vi "HEWH RLT PRAT.vi"() -> ()   [LabVIEW 2016] (continued)
              tunnel: w3221 -> [w3243 _]
              tunnel: w3220 -> [w3244 _]
              tunnel: w3218 -> [w3242 _]
              tunnel: w3217 -> [w3241 _]
              tunnel: w3215 -> [w3239 _]
              tunnel: w3210 -> [w3238 _]
              frame False {
                n1364 = Generate User Event(user event=w3250, event data cluster=TRUE ("event data"), error in=w3249) -> (error out=w3247:errorcluster)  [unwired: 1 in, 1 out]
                n1365 = local write "StationD Setpoint"(w3239) -> ()
                n1366 = local write "Disable Station 4"(HEWH_RLT_Station_Disable."Enable Station" ("Disable Station 4")) -> ()
                n1367 = local write "Cutout Delay D (sec)"(w3241) -> ()
                n1368 = Generate User Event(user event=w3245, event data cluster=TRUE ("event data"), error in=w3247) -> (error out=w3246:errorcluster)  [unwired: 1 in, 1 out]
                "Station D Test Sequence" <- w3253
                "Station ID to Reset" <- w3252
                "Appliance Details D" <- w3244
                "Updated File Path D" <- w3243
                "Log Data Output (D)" <- w3242
                "Test Procedure 4" <- w3238
              }
              frame True {
              }
            }
          }
          event "DAQ for A": Value Change {
            n1369 = event-data() -> ("NewVal"=w3255:bool)  [unwired: 1 in, 5 out]
            n1370 = case shown="True" w3255 {
              frame False {
                w3259 = T67."Enabled" ("Disabled")
                n1371 = property on="DAQ for A" class="Bool (strict)"("DisabledEnum"=w3259) -> ()  [unwired: 2 in, 2 out]
                n1372 = property on="DAQ for B" class="Bool (strict)"("DisabledEnum"=w3259) -> ()  [unwired: 2 in, 2 out]
                n1373 = property on="DAQ for C" class="Bool (strict)"("DisabledEnum"=w3259) -> ()  [unwired: 2 in, 2 out]
                n1374 = property on="DAQ for D" class="Bool (strict)"("DisabledEnum"=w3259) -> ()  [unwired: 2 in, 2 out]
              }
              frame True {
                w3261 = T67."Disabled and Grayed Out" ("Disabled")
                n1375 = property on="DAQ for D" class="Bool (strict)"("DisabledEnum"=w3261) -> ()  [unwired: 2 in, 2 out]
                n1376 = property on="DAQ for B" class="Bool (strict)"("DisabledEnum"=w3261) -> ()  [unwired: 2 in, 2 out]
                n1377 = property on="DAQ for C" class="Bool (strict)"("DisabledEnum"=w3261) -> ()  [unwired: 2 in, 2 out]
                n1378 = property on="DAQ for A" class="Bool (strict)"("DisabledEnum"=T67."Enabled" ("Disabled")) -> ()  [unwired: 2 in, 2 out]
              }
            }
          }
          event "DAQ for B": Value Change {
            n1379 = event-data() -> ("NewVal"=w3262:bool)  [unwired: 1 in, 5 out]
            n1380 = case shown="True" w3262 {
              frame False {
                w3266 = T67."Enabled" ("Disabled")
                n1381 = property on="DAQ for A" class="Bool (strict)"("DisabledEnum"=w3266) -> ()  [unwired: 2 in, 2 out]
                n1382 = property on="DAQ for B" class="Bool (strict)"("DisabledEnum"=w3266) -> ()  [unwired: 2 in, 2 out]
                n1383 = property on="DAQ for C" class="Bool (strict)"("DisabledEnum"=w3266) -> ()  [unwired: 2 in, 2 out]
                n1384 = property on="DAQ for D" class="Bool (strict)"("DisabledEnum"=w3266) -> ()  [unwired: 2 in, 2 out]
              }
              frame True {
                w3267 = T67."Disabled and Grayed Out" ("Disabled")
                n1385 = property on="DAQ for A" class="Bool (strict)"("DisabledEnum"=w3267) -> ()  [unwired: 2 in, 2 out]
                n1386 = property on="DAQ for C" class="Bool (strict)"("DisabledEnum"=w3267) -> ()  [unwired: 2 in, 2 out]
                n1387 = property on="DAQ for D" class="Bool (strict)"("DisabledEnum"=w3267) -> ()  [unwired: 2 in, 2 out]
                n1388 = property on="DAQ for B" class="Bool (strict)"("DisabledEnum"=T67."Enabled" ("Disabled")) -> ()  [unwired: 2 in, 2 out]
              }
            }
          }
          event "DAQ for C": Value Change {
            n1389 = event-data() -> ("NewVal"=w3269:bool)  [unwired: 1 in, 5 out]
            n1390 = case shown="True" w3269 {
              frame False {
                w3273 = T67."Enabled" ("Disabled")
                n1391 = property on="DAQ for A" class="Bool (strict)"("DisabledEnum"=w3273) -> ()  [unwired: 2 in, 2 out]
                n1392 = property on="DAQ for B" class="Bool (strict)"("DisabledEnum"=w3273) -> ()  [unwired: 2 in, 2 out]
                n1393 = property on="DAQ for C" class="Bool (strict)"("DisabledEnum"=w3273) -> ()  [unwired: 2 in, 2 out]
                n1394 = property on="DAQ for D" class="Bool (strict)"("DisabledEnum"=w3273) -> ()  [unwired: 2 in, 2 out]
              }
              frame True {
                w3274 = T67."Disabled and Grayed Out" ("Disabled")
                n1395 = property on="DAQ for A" class="Bool (strict)"("DisabledEnum"=w3274) -> ()  [unwired: 2 in, 2 out]
                n1396 = property on="DAQ for B" class="Bool (strict)"("DisabledEnum"=w3274) -> ()  [unwired: 2 in, 2 out]
                n1397 = property on="DAQ for D" class="Bool (strict)"("DisabledEnum"=w3274) -> ()  [unwired: 2 in, 2 out]
                n1398 = property on="DAQ for C" class="Bool (strict)"("DisabledEnum"=T67."Enabled" ("Disabled")) -> ()  [unwired: 2 in, 2 out]
              }
            }
          }
          event "DAQ for D": Value Change {
            n1399 = event-data() -> ("NewVal"=w3276:bool)  [unwired: 1 in, 5 out]
            n1400 = case shown="True" w3276 {
              frame False {
                w3280 = T67."Enabled" ("Disabled")
                n1401 = property on="DAQ for A" class="Bool (strict)"("DisabledEnum"=w3280) -> ()  [unwired: 2 in, 2 out]
                n1402 = property on="DAQ for B" class="Bool (strict)"("DisabledEnum"=w3280) -> ()  [unwired: 2 in, 2 out]
                n1403 = property on="DAQ for C" class="Bool (strict)"("DisabledEnum"=w3280) -> ()  [unwired: 2 in, 2 out]
                n1404 = property on="DAQ for D" class="Bool (strict)"("DisabledEnum"=w3280) -> ()  [unwired: 2 in, 2 out]
              }
              frame True {
                w3282 = T67."Disabled and Grayed Out" ("Disabled")
                n1405 = property on="DAQ for A" class="Bool (strict)"("DisabledEnum"=w3282) -> ()  [unwired: 2 in, 2 out]
                n1406 = property on="DAQ for B" class="Bool (strict)"("DisabledEnum"=w3282) -> ()  [unwired: 2 in, 2 out]
                n1407 = property on="DAQ for C" class="Bool (strict)"("DisabledEnum"=w3282) -> ()  [unwired: 2 in, 2 out]
                n1408 = property on="DAQ for D" class="Bool (strict)"("DisabledEnum"=T67."Enabled" ("Disabled")) -> ()  [unwired: 2 in, 2 out]
              }
            }
          }
          event "Set Valves": Value Change {
            n1409 = event-data() -> ("NewVal"=w3284:bool)  [unwired: 1 in, 5 out]
            n1410 = call "UTILITY Aquire Semaphore.vi"("error in (no error)"=w3291, "Refnum in"=w3288) -> ("error out"=w3283:errorcluster, "Refnum out"=w3287:T56)  [unwired: 7 in, 1 out]
            n1411 = case shown="True" w3284 {
              tunnel: w3283 -> [w3292 w3299]
              tunnel: [w3292 w3298] -> w3289
              tunnel: w3286 -> [_ w3294]
              frame False {
              }
              frame True {
                n1412 = Unbundle By Name(w3294) -> ("Test Fixture Hardware.Analog Data.Yokogawa.MW100"=w3295:refnum<visa-resource-name>)
                n1413 = local read "Pressurize Tank?"() -> (w3296:bool)
                n1414 = call "HEWH Solenoid Bank.vi"("VISA session"=w3295, "Valve Bank Setting"="Valve Bank Setting", "Station ID"="Station ID", "Pressurize Tank?"=w3296, "Error In"=w3299, "Debug"=TRUE) -> ("Error Out"=w3298:errorcluster)  [unwired: 8 in, 1 out]
              }
            }
            n1415 = call "UTILITY Release Semaphore.vi"("error in (no error)"=w3289, "Refnum in"=w3287) -> ("error out"=w3290:errorcluster)  [unwired: 9 in]
          }
          event "Send GEA CMD": Value Change {
            n1416 = event-data() -> ()  [unwired: 1 in, 6 out]
            n1417 = local read "Station ID"() -> (w3309:T25)
            n1418 = call "HEWH_DSM_CMD.vi"("Heating Mode"="Heating Mode", "GEA2 Commands and Requests"=GEA2_Commands."CMD_UPDATE_MODE") -> ("Input Data"=w3312:T74)  [unwired: 7 in, 1 out]
            n1419 = call "HEWH_DSM_CMD.vi"("Temperature"="Unit Setpoint", "GEA2 Commands and Requests"=GEA2_Commands."CMD_WRITE_SETPOINTS") -> ("Input Data"=w3311:T74)  [unwired: 7 in, 1 out]
            n1420 = case shown="\"A\"" w3309 {
              tunnel: w3313 -> [w3320 w3328 w3347 w3368 w3389]
              tunnel: w3312 -> [_ w3327 w3344 w3365 w3386]
              tunnel: w3311 -> [_ w3324 w3345 w3366 w3387]
              tunnel: [w3320 w3323 w3346 w3367 w3388] -> w3310
              tunnel: w3308 -> [_ _ _ _ w3384]
              tunnel: w3307 -> [_ _ _ _ w3385]
              tunnel: w3306 -> [_ _ _ w3363 _]
              tunnel: w3305 -> [_ _ _ w3364 _]
              tunnel: w3304 -> [_ _ w3343 _ _]
              tunnel: w3303 -> [_ _ w3342 _ _]
              tunnel: w3302 -> [_ w3321 _ _ _]
              tunnel: w3301 -> [_ w3322 _ _ _]
              frame "", Default {
              }
              frame "A" {
                n1421 = for {
                  N: 5 -> [_]
                  tunnel: w3322 -> [w3341]
                  tunnel: w3321 -> [w3340]
                  tunnel: w3327 -> [w3337]
                  shift-right: [w3338] -> w3325
                  shift-left: w3328 -> [w3339]
                  n1422 = call "GEA2 Send and Receive Message.vi"("GEA2 Reference In"=w3341, "Input Data"=w3337, "GEA2 Event Registration"=w3340, "Error In"=w3339) -> ("Error Out"=w3338:errorcluster)  [unwired: 6 in, 5 out]
                  n1423 = Wait Until Next ms Multiple(millisecond multiple=u32 100) -> ()  [unwired: 1 out]
                }
                n1424 = for {
                  N: 5 -> [_]
                  tunnel: w3322 -> [w3335]
                  tunnel: w3321 -> [w3334]
                  tunnel: w3324 -> [w3331]
                  shift-right: [w3332] -> w3323
                  shift-left: w3325 -> [w3333]
                  n1425 = call "GEA2 Send and Receive Message.vi"("GEA2 Reference In"=w3335, "Input Data"=w3331, "GEA2 Event Registration"=w3334, "Error In"=w3333) -> ("Error Out"=w3332:errorcluster)  [unwired: 6 in, 5 out]
                  n1426 = Wait Until Next ms Multiple(millisecond multiple=u32 100) -> ()  [unwired: 1 out]
                }
              }
              frame "B" {
                n1427 = for {
                  N: 5 -> [_]
                  tunnel: w3342 -> [w3362]
                  tunnel: w3343 -> [w3361]
                  tunnel: w3344 -> [w3358]
                  shift-right: [w3359] -> w3348
                  shift-left: w3347 -> [w3360]
                  n1428 = call "GEA2 Send and Receive Message.vi"("GEA2 Reference In"=w3362, "Input Data"=w3358, "GEA2 Event Registration"=w3361, "Error In"=w3360) -> ("Error Out"=w3359:errorcluster)  [unwired: 6 in, 5 out]
                  n1429 = Wait Until Next ms Multiple(millisecond multiple=u32 100) -> ()  [unwired: 1 out]
                }
                n1430 = for {
                  N: 5 -> [_]
                  tunnel: w3342 -> [w3356]
                  tunnel: w3343 -> [w3355]
                  tunnel: w3345 -> [w3352]
                  shift-right: [w3353] -> w3346
                  shift-left: w3348 -> [w3354]
                  n1431 = call "GEA2 Send and Receive Message.vi"("GEA2 Reference In"=w3356, "Input Data"=w3352, "GEA2 Event Registration"=w3355, "Error In"=w3354) -> ("Error Out"=w3353:errorcluster)  [unwired: 6 in, 5 out]
                  n1432 = Wait Until Next ms Multiple(millisecond multiple=u32 100) -> ()  [unwired: 1 out]
                }
              }
              frame "C" {
                n1433 = for {
                  N: 5 -> [_]
                  tunnel: w3364 -> [w3383]
                  tunnel: w3363 -> [w3382]
                  tunnel: w3365 -> [w3379]
                  shift-right: [w3380] -> w3369
                  shift-left: w3368 -> [w3381]
                  n1434 = call "GEA2 Send and Receive Message.vi"("GEA2 Reference In"=w3383, "Input Data"=w3379, "GEA2 Event Registration"=w3382, "Error In"=w3381) -> ("Error Out"=w3380:errorcluster)  [unwired: 6 in, 5 out]
                  n1435 = Wait Until Next ms Multiple(millisecond multiple=u32 100) -> ()  [unwired: 1 out]
                }
                n1436 = for {
                  N: 5 -> [_]
                  tunnel: w3364 -> [w3377]
                  tunnel: w3363 -> [w3376]
                  tunnel: w3366 -> [w3373]
                  shift-right: [w3374] -> w3367
                  shift-left: w3369 -> [w3375]
                  n1437 = call "GEA2 Send and Receive Message.vi"("GEA2 Reference In"=w3377, "Input Data"=w3373, "GEA2 Event Registration"=w3376, "Error In"=w3375) -> ("Error Out"=w3374:errorcluster)  [unwired: 6 in, 5 out]
                  n1438 = Wait Until Next ms Multiple(millisecond multiple=u32 100) -> ()  [unwired: 1 out]
                }
              }
              frame "D" {
                n1439 = for {
                  N: 5 -> [_]
                  tunnel: w3385 -> [w3404]
                  tunnel: w3384 -> [w3403]
                  tunnel: w3386 -> [w3400]
                  shift-right: [w3401] -> w3390
                  shift-left: w3389 -> [w3402]
                  n1440 = call "GEA2 Send and Receive Message.vi"("GEA2 Reference In"=w3404, "Input Data"=w3400, "GEA2 Event Registration"=w3403, "Error In"=w3402) -> ("Error Out"=w3401:errorcluster)  [unwired: 6 in, 5 out]
                  n1441 = Wait Until Next ms Multiple(millisecond multiple=u32 100) -> ()  [unwired: 1 out]
                }
                n1442 = for {
                  N: 5 -> [_]
                  tunnel: w3385 -> [w3398]
                  tunnel: w3384 -> [w3397]
                  tunnel: w3387 -> [w3394]
                  shift-right: [w3395] -> w3388
                  shift-left: w3390 -> [w3396]
                  n1443 = call "GEA2 Send and Receive Message.vi"("GEA2 Reference In"=w3398, "Input Data"=w3394, "GEA2 Event Registration"=w3397, "Error In"=w3396) -> ("Error Out"=w3395:errorcluster)  [unwired: 6 in, 5 out]
                  n1444 = Wait Until Next ms Multiple(millisecond multiple=u32 100) -> ()  [unwired: 1 out]
                }
              }
            }
          }
          event "X-Axis - Station A", "Y-Axis1 - Station A", "Y-Axis2 - Station A": Value Change {
            n1445 = event-data() -> ()  [unwired: 1 in, 6 out]
            n1446 = local read "Station A"() -> (w3409:string[][])
            n1447 = Transpose 2D Array(2D array=w3409) -> (transposed array=w3406:string[][])
            n1448 = Index Array(array=w3406, index (row)=0 ("disabled index (col)")) -> (element=w3412:string[])  [unwired: 1 in]
            n1449 = Index Array(array=w3406, index (row)=0 ("disabled index (col)")) -> (element=w3411:string[])  [unwired: 1 in]
            n1450 = Index Array(array=w3406, index (row)=0 ("disabled index (col)")) -> (element=w3410:string[])  [unwired: 1 in]
            n1451 = property on="X-Axis - Station A" class="CmbBox"("Strings[]"=w3412) -> ()  [unwired: 2 in, 2 out]
            n1452 = property on="Y-Axis2 - Station A" class="CmbBox"("Strings[]"=w3410) -> ()  [unwired: 2 in, 2 out]
            n1453 = property on="Y-Axis1 - Station A" class="CmbBox"("Strings[]"=w3411) -> ()  [unwired: 2 in, 2 out]
          }
          event "Y-Axis1 - Station B", "X-Axis - Station B", "Y-Axis2 - Station B": Value Change {
            n1454 = event-data() -> ()  [unwired: 1 in, 6 out]
            n1455 = local read "Station B"() -> (w3420:string[][])
            n1456 = Transpose 2D Array(2D array=w3420) -> (transposed array=w3419:string[][])
            n1457 = Index Array(array=w3419, index (row)=0 ("disabled index (col)")) -> (element=w3423:string[])  [unwired: 1 in]
            n1458 = Index Array(array=w3419, index (row)=0 ("disabled index (col)")) -> (element=w3422:string[])  [unwired: 1 in]
            n1459 = Index Array(array=w3419, index (row)=0 ("disabled index (col)")) -> (element=w3421:string[])  [unwired: 1 in]
            n1460 = property on="X-Axis - Station B" class="CmbBox"("Strings[]"=w3423) -> ()  [unwired: 2 in, 2 out]
            n1461 = property on="Y-Axis1 - Station B" class="CmbBox"("Strings[]"=w3422) -> ()  [unwired: 2 in, 2 out]
            n1462 = property on="Y-Axis2 - Station B" class="CmbBox"("Strings[]"=w3421) -> ()  [unwired: 2 in, 2 out]
          }
          event "X-Axis - Station C", "Y-Axis1 - Station C", "Y-Axis2 - Station C": Value Change {
            n1463 = event-data() -> ()  [unwired: 1 in, 6 out]
            n1464 = local read "Station C"() -> (w3431:string[][])
            n1465 = Transpose 2D Array(2D array=w3431) -> (transposed array=w3430:string[][])
            n1466 = Index Array(array=w3430, index (row)=0 ("disabled index (col)")) -> (element=w3434:string[])  [unwired: 1 in]
            n1467 = Index Array(array=w3430, index (row)=0 ("disabled index (col)")) -> (element=w3433:string[])  [unwired: 1 in]
            n1468 = Index Array(array=w3430, index (row)=0 ("disabled index (col)")) -> (element=w3432:string[])  [unwired: 1 in]
            n1469 = property on="X-Axis - Station C" class="CmbBox"("Strings[]"=w3434) -> ()  [unwired: 2 in, 2 out]
            n1470 = property on="Y-Axis1 - Station C" class="CmbBox"("Strings[]"=w3433) -> ()  [unwired: 2 in, 2 out]
            n1471 = property on="Y-Axis2 - Station C" class="CmbBox"("Strings[]"=w3432) -> ()  [unwired: 2 in, 2 out]
          }
          event "X-Axis - Station D", "Y-Axis1 - Station D", "Y-Axis2 - Station D": Value Change {
            n1472 = event-data() -> ()  [unwired: 1 in, 6 out]
            n1473 = local read "Station D"() -> (w3441:string[][])
            n1474 = Transpose 2D Array(2D array=w3441) -> (transposed array=w3442:string[][])
            n1475 = Index Array(array=w3442, index (row)=0 ("disabled index (col)")) -> (element=w3445:string[])  [unwired: 1 in]
            n1476 = Index Array(array=w3442, index (row)=0 ("disabled index (col)")) -> (element=w3444:string[])  [unwired: 1 in]
            n1477 = Index Array(array=w3442, index (row)=0 ("disabled index (col)")) -> (element=w3443:string[])  [unwired: 1 in]
            n1478 = property on="X-Axis - Station D" class="CmbBox"("Strings[]"=w3445) -> ()  [unwired: 2 in, 2 out]
            n1479 = property on="Y-Axis1 - Station D" class="CmbBox"("Strings[]"=w3444) -> ()  [unwired: 2 in, 2 out]
            n1480 = property on="Y-Axis2 - Station D" class="CmbBox"("Strings[]"=w3443) -> ()  [unwired: 2 in, 2 out]
          }
          event "Reset Power Analyzer", "Start/Pause test": Value Change {
            n1481 = event-data() -> ("NewVal"=w3449:bool)  [unwired: 1 in, 5 out]
            n1482 = case shown="True" w3449 {
              tunnel: w3451 -> [w3454 w3456]
              tunnel: [w3454 w3455] -> w3450
              frame False {
              }
              frame True {
                n1483 = local read "MW100"() -> (w3457:refnum<visa-resource-name>)
                n1484 = local read "Yokogawa WT210"() -> (w3458:refnum<visa-resource-name>)
                n1485 = local read "Power Analyzer"() -> (w3459:T11)
                n1486 = case shown="\"WT300\"" w3459 {
                  tunnel: w3458 -> [_ w3468]
                  tunnel: w3457 -> [w3460 w3467]
                  tunnel: w3456 -> [w3462 w3466]
                  tunnel: [w3461 w3464] -> w3455
                  frame "", Default {
                    n1487 = call "HEWH Reset MW100.vi"("error in (no error)"=w3462, "MW100 VISA In"=w3460) -> ("error out"=w3461:errorcluster)  [unwired: 8 in, 1 out]
                  }
                  frame "WT300" {
                    n1488 = call "Yokogawa WT300 Series Reset Integrator.vi"("Initialization Routing?"=FALSE, "Error In"=w3466, "VISA Refnum in"=w3468) -> ("Error Out"=w3465:errorcluster)  [unwired: 7 in, 1 out]
                    n1489 = call "HEWH Reset MW100.vi"("error in (no error)"=w3465, "MW100 VISA In"=w3467) -> ("error out"=w3464:errorcluster)  [unwired: 8 in, 1 out]
                  }
                }
              }
            }
          }
          event "Proportioning\nValve": Value Change {
            n1490 = event-data() -> ("NewVal"=w3470:dbl)  [unwired: 1 in, 5 out]
            n1491 = Bundle By Name(cluster=w3472, "User Controls.Proportional Valve"=w3470) -> (w3471:T86)
            n1492 = call <vilib>:"Add State(s) to Queue__jki_lib_state_machine.vi"("State(s) in Front (\"\")"="Adjust Proportional Valve" ("State(s) in Front (\"\")"), "State(s) in (\"\")"=w3473) -> ("States Out"=w3474:string)  [unwired: 13 in]
          }
          event "Hold Intellifaucet Valves": Value Change {
            n1493 = event-data() -> ("NewVal"=w3476:bool)  [unwired: 1 in, 5 out]
            n1494 = Bundle By Name(cluster=w3478, "Hold Valves A"=w3476) -> (w3477:T86)
            n1495 = case shown="True" w3476 {
              tunnel: ["" ("State(s) in Front (\"\")") "Hold Intellifaucet" ("State(s) in Front (\"\")")] -> w3482
              frame False {
              }
              frame True {
              }
            }
            n1496 = call <vilib>:"Add State(s) to Queue__jki_lib_state_machine.vi"("State(s) in Front (\"\")"=w3482, "State(s) in (\"\")"=w3480) -> ("States Out"=w3481:string)  [unwired: 13 in]
          }
          event Panel Close? {
            n1497 = event-data() -> ()  [unwired: 1 in, 1 out]
            n1498 = call <vilib>:"Add State(s) to Queue__jki_lib_state_machine.vi"("State(s) in Front (\"\")"="Start Shutdown\nExit", "State(s) in (\"\")"=w3490) -> ("States Out"=w3489:string)  [unwired: 13 in]
            n1499 = event-data("Discard?"=TRUE) -> ()  [unwired: 1 in, 1 out]
          }
        }
      }
      frame "---------- Core ----------" {
        n1500 = call <vilib>:"Add State(s) to Queue__jki_lib_state_machine.vi"("State(s) in (\"\")"=w3494) -> ("States Out"=w3493:string)  [unwired: 14 in]
      }
      frame Default {
        w3504 = 42 items=["No error", "Argument error", "Memory is full", "Out of zone", "End of file", "File already open", "Generic file I/O error", "File not found", "File permission error", "Disk is full", "Duplicate path", "Too many files open", "System feature not enabled", "Resource file not found", "Cannot add resource", "Resource not found", "Image not found", "Image memory error", "Pen does not exist", "Config type invalid", "Config token not found", "Config parse error", "Config memory error", "Bad external code format", "Bad external code offset", "External code not present", "Null window", "Destroy window error", "Null menu", "Print aborted", "Bad print record", "Print driver error", "Windows error during printing", "Memory error during printing", "Print dialog error", "Generic print error", "Invalid device refnum", "Device not found", "Device parameter error", "Device unit error", "Cannot open device", "Device call aborted", "Generic error", "Cancelled by user", "Object ID too low", "Object ID too high", "Object not in heap", "Unknown heap", "Unknown object (invalid DefProc)", "Unknown object (DefProc not in table)", "Message out of range", "Invalid (null) method", "Unknown message", "Manager call not supported", "Bad address", "Network operation in progress", "Network operation timed out", "Connection is busy", "Network attribute not supported", "Network error", "Address in use", "System out of memory", "Connection aborted", "Connection refused", "Not connected", "Already connected", "Connection closed", "Initialization error (interapplication manager)", "Bad occurrence", "Wait on unbound occurrence handler", "Occurrence queue overflow", "Datalog type conflict", "Unused", "Unrecognized type (interapplication manager)", "Memory corrupt", "Failed to make temporary DLL", "Old CIN version", "Drag socket not found", "Failed to load drop-object", "Failed to register OLE object", "Failed to release OLE object", "Format specifier type mismatch", "Unknown format specifier", "Too few format specifiers", "Too many format specifiers", "Scan failed", "Newer CIN version", "Error converting to variant", "Runtime menu error", "Password tampered", "Variant attribute not found", "Incompatible variant data type", "Event data is not available", "Event Store is not present", "Occurrence is not found", "Event Queue is not created", "Event info is not available", "Refnum passed is NULL", "Error retrieving Class GUID", "Error retrieving CoClass GUID", "Error retrieving TypeLib GUID.", "Bad built application magic bytes.", "Specific driver is different from the specific driver associated with the Logical Name.", "There is no session opened to the class driver.", "Max Error", "MAX - Error with config objects", "MAX - Error loading configuration", "MAX - Group not supported"]
        # "Current State"
        # "Handle mistyped state name (developer tool)"
        n1501 = Format Into String(format string="Software Exception: Unhandled State \"%s\"." ("message"), error in=w3500, w3495) -> (resulting string=w3503:string, error out=w3502:errorcluster)  [unwired: 1 in]
        n1502 = call <vilib>:"Error Cluster From Error Code.vi"("show call chain? (False)"=TRUE, "error in (no error)"=w3502, "error message (\"\")"=w3503, "error code (0)"=w3504) -> ("error out"=w3501:errorcluster)  [unwired: 5 in]
        n1503 = call <vilib>:"Add State(s) to Queue__jki_lib_state_machine.vi"("State(s) in (\"\")"=w3499) -> ("States Out"=w3498:string)  [unwired: 14 in]
      }
      frame "Error Handler" {
        # "Unhandled Error -- Display it"
        # "Clear error"
        n1504 = call <vilib>:"General Error Handler.vi"("error in (no error)"=w3507) -> ()  [unwired: 10 in, 5 out]
        n1505 = call <vilib>:"Add State(s) to Queue__jki_lib_state_machine.vi"("State(s) in Front (\"\")"="/* Post Error States", "State(s) in (\"\")"=w3511) -> ("States Out"=w3510:string)  [unwired: 13 in]
      }
      frame "Exit" {
        n1506 = call <vilib>:"Add State(s) to Queue__jki_lib_state_machine.vi"("State(s) in (\"\")"=w3516) -> ("States Out"=w3515:string)  [unwired: 14 in]
      }
      frame "---------- Data ----------" {
        n1507 = call <vilib>:"Add State(s) to Queue__jki_lib_state_machine.vi"("State(s) in (\"\")"=w3520) -> ("States Out"=w3519:string)  [unwired: 14 in]
      }
      frame "Data: Initialize" {
        # "I use this a a temporary array to build\nall of the cal data"
        n1508 = while {
          tunnel: [w3544] -> w3531
          tunnel: ["User Controls"] -> w3530
          tunnel: [w3542] -> w3529
          tunnel: [w3543] -> w3528
          tunnel: [w3540] -> w3527
          tunnel: [w3539] -> w3525
          tunnel: [w3538] -> w3524
          tunnel: [w3537] -> w3523
          tunnel: [w3536] -> w3522
          tunnel: [w3535] -> w3521
          stop <- w3546 stop-if-true
          w3535 = dbl[][] []  # Cal Build Array
          w3536 = FALSE  # Hold Valves D
          w3537 = FALSE  # Hold Valves C
          w3538 = FALSE  # Hold Valves B
          w3539 = FALSE  # Hold Valves A
          w3543 = T85 {"EEV Over A"=FALSE, "EEV Over B"=FALSE, "EEV Over C"=FALSE, "EEV Over D"=FALSE, "T-Out Over A"=FALSE, "T-Out Over B"=FALSE, "T-Out Over C"=FALSE, "T-Out Over D"=FALSE}  # Alarms
          w3544 = T66 {"Current VI Reference"=refnum, "Close Panel on Exit?"=FALSE}  # Core
          n1509 = Wait Until Next ms Multiple(millisecond multiple=u32 250) -> ()  [unwired: 1 out]
          n1510 = local read "Test Fixture Hardware"() -> (w3542:T47)
          n1511 = local read "Init Complete"() -> (w3546:bool)
          n1512 = local read "LV Program"() -> (w3540:T24)
        }
        n1513 = call <vilib>:"Add State(s) to Queue__jki_lib_state_machine.vi"("State(s) in (\"\")"=w3534) -> ("States Out"=w3533:string)  [unwired: 14 in]
        n1514 = Bundle("Core"=w3531, "User Controls"=w3530, "Test Fixture Hardware"=w3529, "Alarms"=w3528, "LV Program"=w3527, "Hold Valves A"=w3525, "Hold Valves B"=w3524, "Hold Valves C"=w3523, "Hold Valves D"=w3522, "Cal Build Array"=w3521) -> (w3526:T86)  [unwired: 1 in]
      }
      frame "---------- Macro ----------" {
        n1515 = call <vilib>:"Add State(s) to Queue__jki_lib_state_machine.vi"("State(s) in (\"\")"=w3550) -> ("States Out"=w3549:string)  [unwired: 14 in]
      }
      frame "---------- Valve Control ----------" {
        n1516 = call <vilib>:"Add State(s) to Queue__jki_lib_state_machine.vi"("State(s) in (\"\")"=w3554) -> ("States Out"=w3553:string)  [unwired: 14 in]
      }
      frame "Start Shutdown" {
        n1517 = call <vilib>:"Add State(s) to Queue__jki_lib_state_machine.vi"("State(s) in (\"\")"=w3559) -> ("States Out"=w3558:string)  [unwired: 14 in]
        "Shutdown" <- "Macro: Exit"
      }
      frame "Inlet Valve A" {
        n1518 = Unbundle By Name(w3569) -> ("Test Fixture Hardware.Analog Data.Yokogawa.MW100"=w3562:refnum<visa-resource-name>, "User Controls.Valve Ctrl.Inlet Valve A"=w3561:T37, "LV Program"=w3564:T24)
        n1519 = call "UTILITY Aquire Semaphore.vi"("error in (no error)"=w3568, "Refnum in"=w3567) -> ("error out"=w3563:errorcluster, "Refnum out"=w3565:T56)  [unwired: 7 in, 1 out]
        n1520 = case shown="\"HEWH\", \"HEWH RLT\", Default" w3564 {
          tunnel: w3563 -> [w3576 w3581]
          tunnel: w3562 -> [w3575 w3579]
          tunnel: w3561 -> [w3572 w3578]
          tunnel: [w3573 w3580] -> w3560
          frame "HEWH", "HEWH RLT", Default {
            n1521 = call "Solenoid - Fill.vi"("Error In"=w3576, "HEWH MW100 Channel Numbers"=T83 "050", "Input Valve"=w3572, "VISA session"=w3575) -> ("Error Out"=w3573:errorcluster)  [unwired: 6 in, 1 out]
          }
          frame "PRAT" {
            n1522 = call "HEWH PRAT Valves.vi"("error in (no error)"=w3581, "Normally Open Valve"=w3578, "Station ID"=Station_ID_Selector."A", "MW100 In"=w3579) -> ("error out"=w3580:errorcluster)  [unwired: 6 in, 1 out]
          }
        }
        n1523 = call "UTILITY Release Semaphore.vi"("error in (no error)"=w3560, "Refnum in"=w3565) -> ("error out"=w3566:errorcluster)  [unwired: 9 in]
        n1524 = call <vilib>:"Add State(s) to Queue__jki_lib_state_machine.vi"("State(s) in (\"\")"=w3571) -> ("States Out"=w3570:string)  [unwired: 14 in]
      }
      frame "Inlet Valve B" {
        n1525 = Unbundle By Name(w3591) -> ("Test Fixture Hardware.Analog Data.Yokogawa.MW100"=w3586:refnum<visa-resource-name>, "User Controls.Valve Ctrl.Inlet Valve B"=w3585:T37, "LV Program"=w3582:T24)
        n1526 = call "UTILITY Aquire Semaphore.vi"("error in (no error)"=w3590, "Refnum in"=w3589) -> ("error out"=w3584:errorcluster, "Refnum out"=w3587:T56)  [unwired: 7 in, 1 out]
        n1527 = case shown="\"PRAT\"" w3582 {
          tunnel: w3584 -> [w3598 w3603]
          tunnel: w3586 -> [w3597 w3601]
          tunnel: w3585 -> [w3596 w3600]
          tunnel: [w3595 w3602] -> w3583
          frame "HEWH", "HEWH RLT", Default {
            n1528 = call "Solenoid - Fill.vi"("Error In"=w3598, "HEWH MW100 Channel Numbers"=T83 "053", "Input Valve"=w3596, "VISA session"=w3597) -> ("Error Out"=w3595:errorcluster)  [unwired: 6 in, 1 out]
          }
          frame "PRAT" {
            n1529 = call "HEWH PRAT Valves.vi"("error in (no error)"=w3603, "Normally Open Valve"=w3600, "Station ID"=Station_ID_Selector."B", "MW100 In"=w3601) -> ("error out"=w3602:errorcluster)  [unwired: 6 in, 1 out]
          }
        }
        n1530 = call "UTILITY Release Semaphore.vi"("error in (no error)"=w3583, "Refnum in"=w3587) -> ("error out"=w3588:errorcluster)  [unwired: 9 in]
        n1531 = call <vilib>:"Add State(s) to Queue__jki_lib_state_machine.vi"("State(s) in (\"\")"=w3593) -> ("States Out"=w3592:string)  [unwired: 14 in]
      }
      frame "Inlet Valve C" {
        n1532 = Unbundle By Name(w3613) -> ("Test Fixture Hardware.Analog Data.Yokogawa.MW100"=w3608:refnum<visa-resource-name>, "User Controls.Valve Ctrl.Inlet Valve C"=w3605:T37, "LV Program"=w3604:T24)
        n1533 = call "UTILITY Aquire Semaphore.vi"("error in (no error)"=w3612, "Refnum in"=w3611) -> ("error out"=w3607:errorcluster, "Refnum out"=w3609:T56)  [unwired: 7 in, 1 out]
        n1534 = case shown="\"HEWH\", \"HEWH RLT\", Default" w3604 {
          tunnel: w3607 -> [w3620 w3625]
          tunnel: w3608 -> [w3619 w3623]
          tunnel: w3605 -> [w3618 w3622]
          tunnel: [w3617 w3624] -> w3606
          frame "HEWH", "HEWH RLT", Default {
            n1535 = call "Solenoid - Fill.vi"("Error In"=w3620, "HEWH MW100 Channel Numbers"=T83 "057", "Input Valve"=w3618, "VISA session"=w3619) -> ("Error Out"=w3617:errorcluster)  [unwired: 6 in, 1 out]
          }
          frame "PRAT" {
            n1536 = call "HEWH PRAT Valves.vi"("error in (no error)"=w3625, "Normally Open Valve"=w3622, "Station ID"=Station_ID_Selector."C", "MW100 In"=w3623) -> ("error out"=w3624:errorcluster)  [unwired: 6 in, 1 out]
          }
        }
        n1537 = call "UTILITY Release Semaphore.vi"("error in (no error)"=w3606, "Refnum in"=w3609) -> ("error out"=w3610:errorcluster)  [unwired: 9 in]
        n1538 = call <vilib>:"Add State(s) to Queue__jki_lib_state_machine.vi"("State(s) in (\"\")"=w3615) -> ("States Out"=w3614:string)  [unwired: 14 in]
      }
      frame "Inlet Valve D" {
        n1539 = Unbundle By Name(w3635) -> ("Test Fixture Hardware.Analog Data.Yokogawa.MW100"=w3630:refnum<visa-resource-name>, "User Controls.Valve Ctrl.Inlet Valve D"=w3629:T37, "LV Program"=w3628:T24)
        n1540 = call "UTILITY Aquire Semaphore.vi"("error in (no error)"=w3634, "Refnum in"=w3633) -> ("error out"=w3627:errorcluster, "Refnum out"=w3631:T56)  [unwired: 7 in, 1 out]
        n1541 = case shown="\"PRAT\"" w3628 {
          tunnel: w3627 -> [w3642 w3647]
          tunnel: w3630 -> [w3641 w3645]
          tunnel: w3629 -> [w3640 w3644]
          tunnel: [w3639 w3646] -> w3626
          frame "HEWH", "HEWH RLT", Default {
            n1542 = call "Solenoid - Fill.vi"("Error In"=w3642, "HEWH MW100 Channel Numbers"=T83 "060", "Input Valve"=w3640, "VISA session"=w3641) -> ("Error Out"=w3639:errorcluster)  [unwired: 6 in, 1 out]
          }
          frame "PRAT" {
            n1543 = call "HEWH PRAT Valves.vi"("error in (no error)"=w3647, "Normally Open Valve"=w3644, "Station ID"=Station_ID_Selector."D", "MW100 In"=w3645) -> ("error out"=w3646:errorcluster)  [unwired: 6 in, 1 out]
          }
        }
        n1544 = call "UTILITY Release Semaphore.vi"("error in (no error)"=w3626, "Refnum in"=w3631) -> ("error out"=w3632:errorcluster)  [unwired: 9 in]
        n1545 = call <vilib>:"Add State(s) to Queue__jki_lib_state_machine.vi"("State(s) in (\"\")"=w3637) -> ("States Out"=w3636:string)  [unwired: 14 in]
      }
      frame "Drain Valve A" {
        n1546 = Unbundle By Name(w3657) -> ("Test Fixture Hardware.Analog Data.Yokogawa.MW100"=w3656:refnum<visa-resource-name>, "User Controls.Valve Ctrl.Drain Valve A"=w3648:T38)
        n1547 = call "UTILITY Aquire Semaphore.vi"("error in (no error)"=w3655, "Refnum in"=w3650) -> ("error out"=w3654:errorcluster, "Refnum out"=w3651:T56)  [unwired: 7 in, 1 out]
        n1548 = call "Solenoid - DRAIN.vi"("Error In"=w3654, "HEWH MW100 Channel Numbers"=T83 "048", "Drain/Purge Valve"=w3648, "VISA session"=w3656) -> ("Error Out"=w3653:errorcluster)  [unwired: 6 in, 1 out]
        n1549 = call "UTILITY Release Semaphore.vi"("error in (no error)"=w3653, "Refnum in"=w3651) -> ("error out"=w3652:errorcluster)  [unwired: 9 in]
        n1550 = call <vilib>:"Add State(s) to Queue__jki_lib_state_machine.vi"("State(s) in (\"\")"=w3659) -> ("States Out"=w3658:string)  [unwired: 14 in]
      }
      frame "Drain Valve B" {
        n1551 = Unbundle By Name(w3669) -> ("Test Fixture Hardware.Analog Data.Yokogawa.MW100"=w3667:refnum<visa-resource-name>, "User Controls.Valve Ctrl.Drain Valve B"=w3668:T38)
        n1552 = call "UTILITY Aquire Semaphore.vi"("error in (no error)"=w3666, "Refnum in"=w3664) -> ("error out"=w3665:errorcluster, "Refnum out"=w3661:T56)  [unwired: 7 in, 1 out]
        n1553 = call "Solenoid - DRAIN.vi"("Error In"=w3665, "HEWH MW100 Channel Numbers"=T83 "051", "Drain/Purge Valve"=w3668, "VISA session"=w3667) -> ("Error Out"=w3663:errorcluster)  [unwired: 6 in, 1 out]
        n1554 = call "UTILITY Release Semaphore.vi"("error in (no error)"=w3663, "Refnum in"=w3661) -> ("error out"=w3662:errorcluster)  [unwired: 9 in]
        n1555 = call <vilib>:"Add State(s) to Queue__jki_lib_state_machine.vi"("State(s) in (\"\")"=w3671) -> ("States Out"=w3670:string)  [unwired: 14 in]
      }
      frame "Drain Valve C" {
        n1556 = Unbundle By Name(w3681) -> ("Test Fixture Hardware.Analog Data.Yokogawa.MW100"=w3679:refnum<visa-resource-name>, "User Controls.Valve Ctrl.Drain Valve C"=w3680:T38)
        n1557 = call "UTILITY Aquire Semaphore.vi"("error in (no error)"=w3678, "Refnum in"=w3676) -> ("error out"=w3677:errorcluster, "Refnum out"=w3673:T56)  [unwired: 7 in, 1 out]
        n1558 = call "Solenoid - DRAIN.vi"("Error In"=w3677, "HEWH MW100 Channel Numbers"=T83 "054", "Drain/Purge Valve"=w3680, "VISA session"=w3679) -> ("Error Out"=w3675:errorcluster)  [unwired: 6 in, 1 out]
        n1559 = call "UTILITY Release Semaphore.vi"("error in (no error)"=w3675, "Refnum in"=w3673) -> ("error out"=w3674:errorcluster)  [unwired: 9 in]
        n1560 = call <vilib>:"Add State(s) to Queue__jki_lib_state_machine.vi"("State(s) in (\"\")"=w3683) -> ("States Out"=w3682:string)  [unwired: 14 in]
      }
      frame "Drain Valve D" {
        n1561 = Unbundle By Name(w3693) -> ("Test Fixture Hardware.Analog Data.Yokogawa.MW100"=w3691:refnum<visa-resource-name>, "User Controls.Valve Ctrl.Drain Valve D"=w3692:T38)
        n1562 = call "UTILITY Aquire Semaphore.vi"("error in (no error)"=w3690, "Refnum in"=w3688) -> ("error out"=w3689:errorcluster, "Refnum out"=w3687:T56)  [unwired: 7 in, 1 out]
        n1563 = call "Solenoid - DRAIN.vi"("Error In"=w3689, "HEWH MW100 Channel Numbers"=T83 "058", "Drain/Purge Valve"=w3692, "VISA session"=w3691) -> ("Error Out"=w3686:errorcluster)  [unwired: 6 in, 1 out]
        n1564 = call "UTILITY Release Semaphore.vi"("error in (no error)"=w3686, "Refnum in"=w3687) -> ("error out"=w3685:errorcluster)  [unwired: 9 in]
        n1565 = call <vilib>:"Add State(s) to Queue__jki_lib_state_machine.vi"("State(s) in (\"\")"=w3695) -> ("States Out"=w3694:string)  [unwired: 14 in]
      }
      frame "Outlet Valve A" {
        n1566 = Unbundle By Name(w3705) -> ("Test Fixture Hardware.Analog Data.Yokogawa.MW100"=w3704:refnum<visa-resource-name>, "User Controls.Valve Ctrl.Outlet Valve A"=w3696:T37)
        n1567 = call "UTILITY Aquire Semaphore.vi"("error in (no error)"=w3703, "Refnum in"=w3701) -> ("error out"=w3702:errorcluster, "Refnum out"=w3698:T56)  [unwired: 7 in, 1 out]
        n1568 = call "HEWH Solenoid Output Set.vi"("Error In"=w3702, "HEWH MW100 Channel Numbers"=T83 "049", "Outlet Valve"=w3696, "VISA session"=w3704) -> ("Error Out"=w3700:errorcluster)  [unwired: 6 in, 1 out]
        n1569 = call "UTILITY Release Semaphore.vi"("error in (no error)"=w3700, "Refnum in"=w3698) -> ("error out"=w3699:errorcluster)  [unwired: 9 in]
        n1570 = call <vilib>:"Add State(s) to Queue__jki_lib_state_machine.vi"("State(s) in (\"\")"=w3707) -> ("States Out"=w3706:string)  [unwired: 14 in]
      }
      frame "Outlet Valve B" {
        n1571 = Unbundle By Name(w3717) -> ("Test Fixture Hardware.Analog Data.Yokogawa.MW100"=w3715:refnum<visa-resource-name>, "User Controls.Valve Ctrl.Outlet Valve B"=w3716:T37)
        n1572 = call "UTILITY Aquire Semaphore.vi"("error in (no error)"=w3714, "Refnum in"=w3713) -> ("error out"=w3712:errorcluster, "Refnum out"=w3709:T56)  [unwired: 7 in, 1 out]
        n1573 = call "HEWH Solenoid Output Set.vi"("Error In"=w3712, "HEWH MW100 Channel Numbers"=T83 "052", "Outlet Valve"=w3716, "VISA session"=w3715) -> ("Error Out"=w3711:errorcluster)  [unwired: 6 in, 1 out]
        n1574 = call "UTILITY Release Semaphore.vi"("error in (no error)"=w3711, "Refnum in"=w3709) -> ("error out"=w3710:errorcluster)  [unwired: 9 in]
        n1575 = call <vilib>:"Add State(s) to Queue__jki_lib_state_machine.vi"("State(s) in (\"\")"=w3719) -> ("States Out"=w3718:string)  [unwired: 14 in]
      }
      frame "Outlet Valve C" {
        n1576 = Unbundle By Name(w3729) -> ("Test Fixture Hardware.Analog Data.Yokogawa.MW100"=w3727:refnum<visa-resource-name>, "User Controls.Valve Ctrl.Outlet Valve C"=w3728:T37)
        n1577 = call "UTILITY Aquire Semaphore.vi"("error in (no error)"=w3726, "Refnum in"=w3722) -> ("error out"=w3725:errorcluster, "Refnum out"=w3721:T56)  [unwired: 7 in, 1 out]
        n1578 = call "HEWH Solenoid Output Set.vi"("Error In"=w3725, "HEWH MW100 Channel Numbers"=T83 "055", "Outlet Valve"=w3728, "VISA session"=w3727) -> ("Error Out"=w3724:errorcluster)  [unwired: 6 in, 1 out]
        n1579 = call "UTILITY Release Semaphore.vi"("error in (no error)"=w3724, "Refnum in"=w3721) -> ("error out"=w3723:errorcluster)  [unwired: 9 in]
        n1580 = call <vilib>:"Add State(s) to Queue__jki_lib_state_machine.vi"("State(s) in (\"\")"=w3731) -> ("States Out"=w3730:string)  [unwired: 14 in]
      }
      frame "Outlet Valve D" {
        n1581 = Unbundle By Name(w3741) -> ("Test Fixture Hardware.Analog Data.Yokogawa.MW100"=w3740:refnum<visa-resource-name>, "User Controls.Valve Ctrl.Outlet Valve D"=w3739:T37)
        n1582 = call "UTILITY Aquire Semaphore.vi"("error in (no error)"=w3738, "Refnum in"=w3737) -> ("error out"=w3736:errorcluster, "Refnum out"=w3733:T56)  [unwired: 7 in, 1 out]
        n1583 = call "HEWH Solenoid Output Set.vi"("Error In"=w3736, "HEWH MW100 Channel Numbers"=T83 "059", "Outlet Valve"=w3739, "VISA session"=w3740) -> ("Error Out"=w3735:errorcluster)  [unwired: 6 in, 1 out]
        n1584 = call "UTILITY Release Semaphore.vi"("error in (no error)"=w3735, "Refnum in"=w3733) -> ("error out"=w3734:errorcluster)  [unwired: 9 in]
        n1585 = call <vilib>:"Add State(s) to Queue__jki_lib_state_machine.vi"("State(s) in (\"\")"=w3743) -> ("States Out"=w3742:string)  [unwired: 14 in]
      }
      frame "Main Power" {
        n1586 = call "UTILITY Aquire Semaphore.vi"("error in (no error)"=w3754, "Refnum in"=w3752) -> ("error out"=w3753:errorcluster, "Refnum out"=w3749:T56)  [unwired: 7 in, 1 out]
        n1587 = Unbundle By Name(w3755) -> ("Test Fixture Hardware.Analog Data.Yokogawa.MW100"=w3756:refnum<visa-resource-name>, "User Controls.Main Power Control"=w3745:bool)
        n1588 = case shown="False" w3745 {
          tunnel: [T37 "ON" ("Normally Open Valve") T37 "OFF" ("Normally Open Valve")] -> w3744
          frame False {
          }
          frame True {
          }
        }
        n1589 = call "INTELLIFAUCET DO Control.vi"("VISA session"=w3756, "Normally Closed Valve?"=FALSE, "HEWH MW100 Channel Numbers"=T83 "047", "Normally Open Valve"=w3744, "Error In"=w3753) -> ("Power ON"=→"Power ON":bool, "error out"=w3751:errorcluster)  [unwired: 7 in, 2 out]
        n1590 = call <vilib>:"Add State(s) to Queue__jki_lib_state_machine.vi"("State(s) in (\"\")"=w3758) -> ("States Out"=w3757:string)  [unwired: 14 in]
        n1591 = call "UTILITY Release Semaphore.vi"("error in (no error)"=w3751, "Refnum in"=w3749) -> ("error out"=w3750:errorcluster)  [unwired: 9 in]
      }
      frame "--------Intellifaucet Control------" {
        n1592 = call <vilib>:"Add State(s) to Queue__jki_lib_state_machine.vi"("State(s) in (\"\")"=w3764) -> ("States Out"=w3763:string)  [unwired: 14 in]
      }
      frame "Start Intellifaucet" {
        n1593 = Unbundle By Name(w3773) -> ("Test Fixture Hardware.Analog Data.Yokogawa.MW100"=w3775:refnum<visa-resource-name>)
        n1594 = call "UTILITY Aquire Semaphore.vi"("error in (no error)"=w3769, "Refnum in"=w3767) -> ("error out"=w3768:errorcluster, "Refnum out"=w3766:T56)  [unwired: 7 in, 1 out]
        n1595 = call "YKMW100 Receive String-clear buff.vi"("VISA session"=w3775, "Timeout (25000)"=u32 500, "error in (no error)"=w3768) -> ("dup VISA session"=w3774:refnum<visa-resource-name>, "error out"=w3771:errorcluster)  [unwired: 10 in, 1 out]
        n1596 = call "UTILITY Release Semaphore.vi"("error in (no error)"=w3771, "Refnum in"=w3766) -> ("error out"=w3770:errorcluster)  [unwired: 9 in]
        n1597 = call "INTELLIFAUCET Driver.vi"("VISA session"=w3774, "Mode"=INTELLIFAUCET_Set_Mode."Start Flow", "Error In"=w3770, "Refnum in"=w3767, "Use Proportion Valve"=FALSE) -> ("Error Out"=w3772:errorcluster)  [unwired: 7 in, 3 out]
        n1598 = call <vilib>:"Add State(s) to Queue__jki_lib_state_machine.vi"("State(s) in (\"\")"=w3779) -> ("States Out"=w3778:string)  [unwired: 14 in]
      }
      frame "Stop Intellifaucet" {
        w3788 = 0.0 ("Target")
        n1599 = Unbundle By Name(w3797) -> ("Test Fixture Hardware.Analog Data.Yokogawa.MW100"=w3789:refnum<visa-resource-name>)
        n1600 = call "UTILITY Aquire Semaphore.vi"("error in (no error)"=w3787, "Refnum in"=w3785) -> ("error out"=w3786:errorcluster, "Refnum out"=w3782:T56)  [unwired: 7 in, 1 out]
        n1601 = call "YKMW100 Receive String-clear buff.vi"("VISA session"=w3789, "Timeout (25000)"=u32 500, "error in (no error)"=w3786) -> ("dup VISA session"=w3795:refnum<visa-resource-name>, "error out"=w3784:errorcluster)  [unwired: 10 in, 1 out]
        n1602 = call "UTILITY Release Semaphore.vi"("error in (no error)"=w3784, "Refnum in"=w3782) -> ("error out"=w3783:errorcluster)  [unwired: 9 in]
        n1603 = call "INTELLIFAUCET Driver.vi"("VISA session"=w3795, "Mode"=INTELLIFAUCET_Set_Mode."Stop Flow", "Error In"=w3783, "Refnum in"=w3785, "Use Proportion Valve"=FALSE) -> ("VISA session out"=w3790:refnum<visa-resource-name>, "Error Out"=w3792:errorcluster)  [unwired: 7 in, 2 out]
        n1604 = call <vilib>:"Add State(s) to Queue__jki_lib_state_machine.vi"("State(s) in (\"\")"=w3800) -> ("States Out"=w3799:string)  [unwired: 14 in]
        n1605 = local write "Proportioning\nValve"(w3788) -> ()
        n1606 = call "PROPORTIONING VALVE MicroAmp Set.vi"("Refnum in"=w3785, "milliseconds to wait"=u32 100, "Debug"=FALSE, "Use Micro Amp Set"=FALSE, "error in (no error)"=w3792, "Target"=w3788, "VISA Refnum in"=w3790) -> ("error out"=w3791:errorcluster)  [unwired: 3 in, 1 out]
      }
      frame "Adjust Temp" {
        # "Operate this on Approx Values\n(Dont wire the 2D Array)"
        n1607 = Unbundle By Name(w3805) -> ("Test Fixture Hardware.Analog Data.Yokogawa.MW100"=w3806:refnum<visa-resource-name>, "User Controls.Intellifaucet \nTemperature"=w3808:dbl)
        n1608 = call "INTELLIFAUCET Driver.vi"("VISA session"=w3806, "Mode"=INTELLIFAUCET_Set_Mode."Adjust Temp", "Use General Conversion"=TRUE, "Temperature(F)"=w3808, "Error In"=w3803, "Refnum in"=w3802) -> ("Error Out"=w3804:errorcluster)  [unwired: 6 in, 3 out]
        n1609 = call <vilib>:"Add State(s) to Queue__jki_lib_state_machine.vi"("State(s) in (\"\")"=w3810) -> ("States Out"=w3809:string)  [unwired: 14 in]
      }
      frame "Adjust Flow" {
        # "Operate this on Approx Values\n(Dont wire the 2D Array)"
        n1610 = Unbundle By Name(w3815) -> ("Test Fixture Hardware.Analog Data.Yokogawa.MW100"=w3817:refnum<visa-resource-name>, "User Controls.Percent Flow"=w3818:dbl)
        n1611 = call "INTELLIFAUCET Driver.vi"("VISA session"=w3817, "Mode"=INTELLIFAUCET_Set_Mode."Adjust Flow", "Use General Conversion"=TRUE, "Flow Rate (GPM)"=w3818, "Error In"=w3813, "Refnum in"=w3812) -> ("Error Out"=w3814:errorcluster)  [unwired: 6 in, 3 out]
        n1612 = call <vilib>:"Add State(s) to Queue__jki_lib_state_machine.vi"("State(s) in (\"\")"=w3820) -> ("States Out"=w3819:string)  [unwired: 14 in]
      }
      frame "Adjust Proportional Valve" {
        n1613 = Unbundle By Name(w3829) -> ("Test Fixture Hardware.Analog Data.Yokogawa.MW100"=w3824:refnum<visa-resource-name>, "User Controls.Proportional Valve"=w3822:dbl)
        n1614 = call "PROPORTIONING VALVE MicroAmp Set.vi"("Refnum in"=w3825, "milliseconds to wait"=u32 100, "Debug"=FALSE, "Use Micro Amp Set"=FALSE, "error in (no error)"=w3827, "Target"=w3822, "VISA Refnum in"=w3824) -> ("error out"=w3826:errorcluster)  [unwired: 3 in, 1 out]
        n1615 = call <vilib>:"Add State(s) to Queue__jki_lib_state_machine.vi"("State(s) in (\"\")"=w3831) -> ("States Out"=w3830:string)  [unwired: 14 in]
      }
      frame "Hold Intellifaucet" {
        n1616 = Unbundle By Name(w3833) -> ("Test Fixture Hardware.Analog Data.Yokogawa.MW100"=w3836:refnum<visa-resource-name>)
        n1617 = call "INTELLIFAUCET Driver.vi"("VISA session"=w3836, "Mode"=INTELLIFAUCET_Set_Mode."Hold", "Error In"=w3835, "Refnum in"=w3832) -> ("Error Out"=w3834:errorcluster)  [unwired: 8 in, 3 out]
        n1618 = call <vilib>:"Add State(s) to Queue__jki_lib_state_machine.vi"("State(s) in (\"\")"=w3839) -> ("States Out"=w3838:string)  [unwired: 14 in]
      }
      frame "---------Alarms Control---------" {
      }
      frame "EEV Test" {
        w3865 = "\"EEV Position (0-480)\"" ("Element")
        # "\"Or\" current alarm status with previous alarm status so that alarm will stay on until cleared"
        # "Check if EEV is over defined limit.\nThis will go into Data Processing Loop once that loop is ready to run fully"
        n1619 = Unbundle By Name(w3850) -> ("Alarms.EEV Over A"=w3849:bool, "Alarms.EEV Over B"=w3847:bool, "Alarms.EEV Over C"=w3848:bool, "Alarms.EEV Over D"=w3846:bool)
        n1620 = local read "Station A"() -> (w3855:string[][])
        n1621 = local read "Station C"() -> (w3853:string[][])
        n1622 = local read "Station B"() -> (w3854:string[][])
        n1623 = local read "Station D"() -> (w3852:string[][])
        n1624 = call "DWE Search 2D Array (String).vi"("Element"=w3865, "Array"=w3852) -> ("element"=w3861:string)  [unwired: 8 in, 1 out]
        n1625 = call "DWE Search 2D Array (String).vi"("Element"=w3865, "Array"=w3853) -> ("element"=w3860:string)  [unwired: 8 in, 1 out]
        n1626 = call "DWE Search 2D Array (String).vi"("Element"=w3865, "Array"=w3854) -> ("element"=w3859:string)  [unwired: 8 in, 1 out]
        n1627 = call "DWE Search 2D Array (String).vi"("Element"=w3865, "Array"=w3855) -> ("element"=w3857:string)  [unwired: 8 in, 1 out]
        n1628 = Decimal String To Number(string=w3861) -> (number=w3864:i32)  [unwired: 2 in, 1 out]
        n1629 = Decimal String To Number(string=w3860) -> (number=w3863:i32)  [unwired: 2 in, 1 out]
        n1630 = Decimal String To Number(string=w3859) -> (number=w3862:i32)  [unwired: 2 in, 1 out]
        n1631 = Decimal String To Number(string=w3857) -> (number=w3858:i32)  [unwired: 2 in, 1 out]
        n1632 = Greater Or Equal?(x=w3864, y="EEV Limit") -> (x >= y?=w3870:bool)
        n1633 = Greater Or Equal?(x=w3862, y="EEV Limit") -> (x >= y?=w3868:bool)
        n1634 = Greater Or Equal?(x=w3863, y="EEV Limit") -> (x >= y?=w3869:bool)
        n1635 = Greater Or Equal?(x=w3858, y="EEV Limit") -> (x >= y?=w3867:bool)
        n1636 = Or(x=w3868, y=w3847) -> (x .or. y?=w3872:bool)
        "EEV Over B" <- w3872
        n1637 = Or(x=w3869, y=w3848) -> (x .or. y?=w3873:bool)
        "EEV Over C" <- w3873
        n1638 = Or(x=w3870, y=w3846) -> (x .or. y?=w3874:bool)
        "EEV Over D" <- w3874
        n1639 = Or(x=w3867, y=w3849) -> (x .or. y?=w3871:bool)
        "EEV Over A" <- w3871
        n1640 = Compound Arithmetic op=OR(w3871, w3872, w3873, w3874) -> (w3866:bool)
        n1641 = case shown="False" w3866 {
          frame False {
            # "No error"
            n1642 = property on="EEV Limit" class="DigNum (strict)"("NumText.BG Color"=u32 6618880 ("Color Box")) -> ()  [unwired: 2 in, 2 out]
          }
          frame True {
            # "Error"
            n1643 = property on="EEV Limit" class="DigNum (strict)"("NumText.BG Color"=u32 16711680 ("Color Box")) -> ()  [unwired: 2 in, 2 out]
          }
        }
        n1644 = Bundle By Name(cluster=w3850, "Alarms.EEV Over A"=w3871, "Alarms.EEV Over B"=w3872, "Alarms.EEV Over C"=w3873, "Alarms.EEV Over D"=w3874) -> (w3843:T86)
        n1645 = call <vilib>:"Add State(s) to Queue__jki_lib_state_machine.vi"("State(s) in (\"\")"=w3845) -> ("States Out"=w3844:string)  [unwired: 14 in]
      }
      frame "Thermal Limits Test" {
        # "This will go into Data Processing Loop once that loop is ready to run fully"
        # "Alarm is set if EEV or T-OUT is over limit"
        n1646 = Unbundle By Name(w3884) -> ("Alarms.T-Out Over A"=w3880:bool, "Alarms.T-Out Over B"=w3879:bool, "Alarms.T-Out Over C"=w3878:bool, "Alarms.T-Out Over D"=w3877:bool)
        n1647 = local read "Station A"() -> (w3889:string[][])
        n1648 = local read "Station C"() -> (w3887:string[][])
        n1649 = local read "Station B"() -> (w3888:string[][])
        n1650 = local read "Station D"() -> (w3886:string[][])
        n1651 = call "DWE Search 2D Array (String).vi"("Element"="T4 - OUT", "Array"=w3886) -> ("element"=w3901:string)  [unwired: 8 in, 1 out]
        n1652 = call "DWE Search 2D Array (String).vi"("Element"="T3 - OUT", "Array"=w3887) -> ("element"=w3900:string)  [unwired: 8 in, 1 out]
        n1653 = call "DWE Search 2D Array (String).vi"("Element"="T1 - OUT", "Array"=w3889) -> ("element"=w3898:string)  [unwired: 8 in, 1 out]
        n1654 = call "DWE Search 2D Array (String).vi"("Element"="T2 - OUT", "Array"=w3888) -> ("element"=w3899:string)  [unwired: 8 in, 1 out]
        n1655 = Fract/Exp String To Number(string=w3901) -> (number=w3893:dbl)  [unwired: 3 in, 1 out]
        n1656 = Fract/Exp String To Number(string=w3900) -> (number=w3892:dbl)  [unwired: 3 in, 1 out]
        n1657 = Fract/Exp String To Number(string=w3898) -> (number=w3890:dbl)  [unwired: 3 in, 1 out]
        n1658 = Fract/Exp String To Number(string=w3899) -> (number=w3891:dbl)  [unwired: 3 in, 1 out]
        n1659 = Greater Or Equal?(x=w3893, y="Thermal Limit") -> (x >= y?=w3916:bool)
        n1660 = Greater Or Equal?(x=w3892, y="Thermal Limit") -> (x >= y?=w3915:bool)
        n1661 = Greater Or Equal?(x=w3890, y="Thermal Limit") -> (x >= y?=w3913:bool)
        n1662 = Greater Or Equal?(x=w3891, y="Thermal Limit") -> (x >= y?=w3914:bool)
        n1663 = Or(x=w3916, y=w3877) -> (x .or. y?=w3921:bool)
        "T-OUT Over D" <- w3921
        n1664 = Or(x=w3915, y=w3878) -> (x .or. y?=w3920:bool)
        "T-OUT Over C" <- w3920
        n1665 = Or(x=w3914, y=w3879) -> (x .or. y?=w3919:bool)
        "T-OUT Over B" <- w3919
        n1666 = Or(x=w3913, y=w3880) -> (x .or. y?=w3918:bool)
        "T-OUT Over A" <- w3918
        n1667 = local read "EEV Over A"() -> (w3903:bool)
        n1668 = local read "EEV Over C"() -> (w3905:bool)
        n1669 = local read "EEV Over B"() -> (w3904:bool)
        n1670 = local read "EEV Over D"() -> (w3906:bool)
        n1671 = Compound Arithmetic op=OR(w3918, w3919, w3920, w3921) -> (w3902:bool)
        n1672 = Or(x=w3918, y=w3903) -> (x .or. y?=w3908:bool)
        n1673 = Or(x=w3921, y=w3906) -> (x .or. y?=w3911:bool)
        n1674 = Or(x=w3920, y=w3905) -> (x .or. y?=w3910:bool)
        n1675 = Or(x=w3919, y=w3904) -> (x .or. y?=w3909:bool)
        n1676 = case shown="False" w3902 {
          frame False {
            n1677 = property on="Thermal Limit" class="DigNum (strict)"("NumText.BG Color"=u32 6618880 ("Color Box")) -> ()  [unwired: 2 in, 2 out]
          }
          frame True {
            n1678 = property on="Thermal Limit" class="DigNum (strict)"("NumText.BG Color"=u32 16711680 ("Color Box")) -> ()  [unwired: 2 in, 2 out]
          }
        }
        n1679 = local write "Alarm A"(w3908) -> ()
        n1680 = local write "Alarm D"(w3911) -> ()
        n1681 = local write "Alarm B"(w3909) -> ()
        n1682 = local write "Alarm C"(w3910) -> ()
